vi "Read_MessageCriticity.vi"(8 "error in (no error)":errorcluster, 11 "Messages in":refnum<class "Messages.lvclass">) -> (0 "error out":errorcluster, 2 "Criticity":T1, 3 "Messages out":refnum<class "Messages.lvclass">)   [LabVIEW 2013, in "Messages.lvclass"]
uses:
  Messages.lvclass
  030 - EVENTS/03 - ToMessageHandlerProcess/enumMessageCriticity.ctl
  Messages.lvclass/Messages.ctl
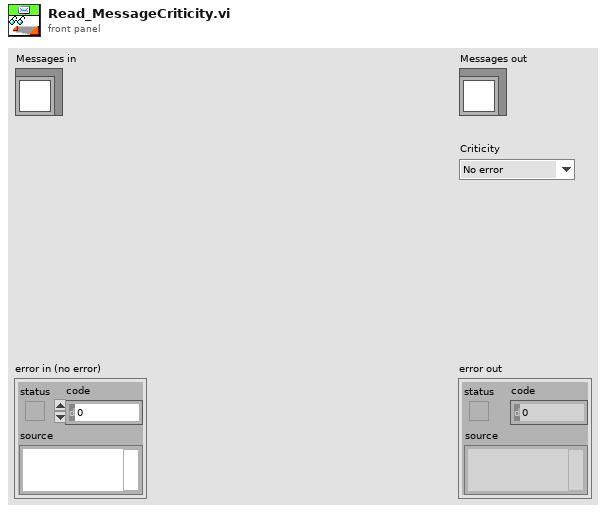
[diagram p1: front panel]
types:
  T1 = typedef "enumMessageCriticity.ctl" = enum16{"No error", "Info", "Warning", "Error", "Fatal error"}
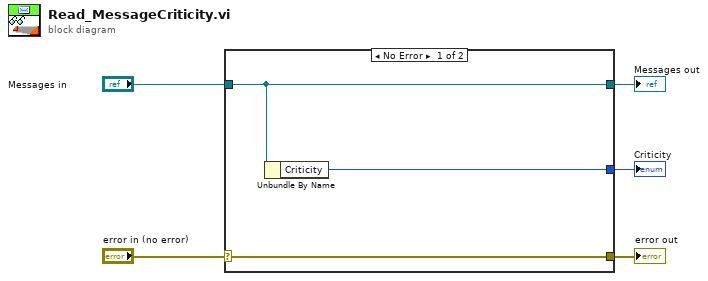
[diagram p0: block diagram]
diagram:
  n1 = case shown="No Error" "error in (no error)" {
    selector: "error in (no error)" -> [w8 w9]
    tunnel: [w8 w9] -> w4
    tunnel: [w7 w10] -> w2
    tunnel: "Messages in" -> [w7 w10]
    tunnel: [w6 _] -> w1
    frame No Error {
      n2 = Unbundle By Name(w7) -> ("Criticity"=w6:T1)
    }
    frame Error {
    }
  }
  "error out" <- w4
  "Messages out" <- w2
  "Criticity" <- w1
